vi "Read Event.vi"(8 "error in (no error)":errorcluster, 11 "Schedule Builder in":refnum<class "Schedule Builder.lvclass">) -> (0 "error out":errorcluster, 2 "Event":refnum<user-event>, 3 "Schedule Builder out":refnum<class "Schedule Builder.lvclass">)   [LabVIEW 2012, in "Schedule Builder.lvclass"]
uses:
  Schedule Builder.lvclass
  Type Defs/Mode Select.ctl
  Schedule Builder.lvclass/Schedule Builder.ctl
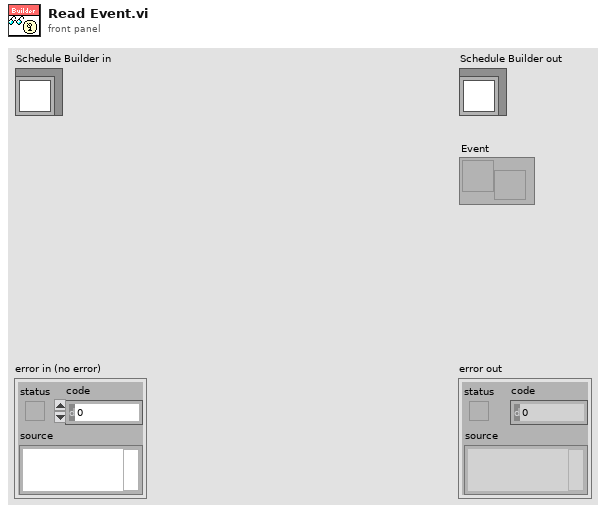
[diagram p1: front panel]
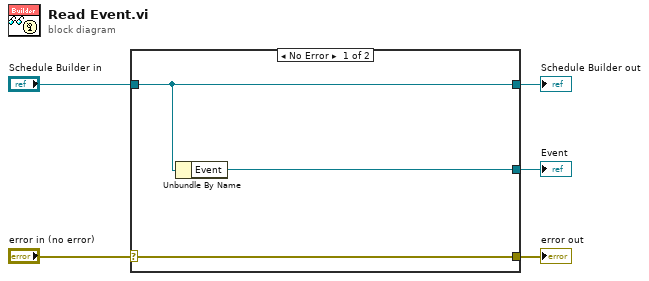
[diagram p0: block diagram]
diagram:
  n1 = case shown="No Error" "error in (no error)" {
    selector: "error in (no error)" -> [w8 w9]
    tunnel: [w8 w9] -> w4
    tunnel: [w7 w10] -> w2
    tunnel: "Schedule Builder in" -> [w7 w10]
    tunnel: [w6 _] -> w1
    frame No Error {
      n2 = Unbundle By Name(w7) -> ("Event"=w6:refnum<user-event>)
    }
    frame Error {
    }
  }
  "error out" <- w4
  "Schedule Builder out" <- w2
  "Event" <- w1
